vi "DMA-Ch.vi"(4 "DMATtoHOST":refnum<k21>="DMATtoHOST0", 6 "ProcessingFIFO":refnum<k21>="Processing0", 7 "IntermediateFIFO":refnum<k21>="FIFO0", 8 "Processing":bool, 10 "Source Name":refnum<k21>="100 MHz Clock", 11 "DMA number":i16) -> ()   [LabVIEW 2013]
uses:
  ctl.ctl
  StateControl.ctl
  <vilib>/Platform/TimedLoop/XDataNode/timing_clust.ctl
  <vilib>/Platform/TimedLoop/XDataNode/nitl_modes.ctl
  <vilib>/Platform/TimedLoop/XDataNode/wakeup.ctl
  N Channels.ctl
  <vilib>/rvi/Emulation/niFpgaSctlEmulationGetInTimedLoop.vi
  <vilib>/rvi/Emulation/niFpgaEmulationReportErrorSimple.vi
  <vilib>/rvi/Emulation/niFpgaGetClockAttributes.vi
  <vilib>/rvi/Emulation/niFpgaCriticalErrorInLSC.vi
  <vilib>/rvi/DataTransferAndStorage/Container/Common/niFpgaContainerExecOnDevCompGetState.vi
  <vilib>/rvi/FIFO/Fifo_Resource/nirvififoEmulationGetNumberOfElementsToReadFpgaImpl.vi
  <vilib>/rvi/DataTransferAndStorage/Container/Common/niFpgaContainerGetUniqueNameForEmu.vi
  <vilib>/rvi/interface/RandomDataEmulation/nirviRandomDataFPGAFIFO.vi
  <vilib>/rvi/interface/RandomDataEmulation/niFpgaRandomDataHandleErrors.vi
  <vilib>/rvi/eio/common/nirviEmuReportErrorAndStop.vi
  <vilib>/rvi/FIFO/Fifo_Resource/nirvififoEmulationReadFpgaImpl.vi
  <vilib>/rvi/FIFO/Fifo_Resource/nirvififoEmulationWriteFpgaImpl.vi
  <vilib>/rvi/Emulation/niFpgaProcessEmulError.vi
  GlobalReg.vi
  <vilib>/Platform/TimedLoop/XDataNode/XDataNode.xnode
  <vilib>/rvi/DataTransferAndStorage/Container/XNode/niFpgaContainer.xnode
  <vilib>/rvi/FIFO/Fifo_Resource/niFpgaFifoEmulationRefIn.vi
  <vilib>/rvi/interface/RandomDataEmulation/nirviRandomDataFpgaReadWriteTemplate.vi
  <vilib>/Platform/TimedLoop/XDataNode/XDNodeRunTimeDep.lvlib
panel:
  in  "Cluster in":T1
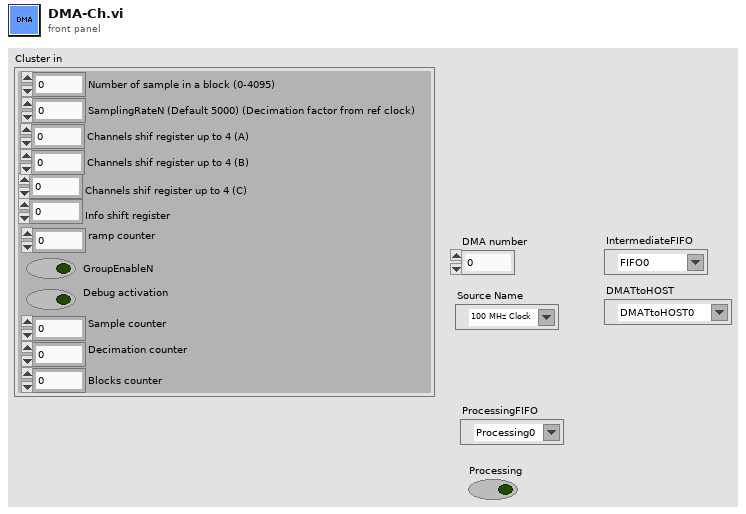
[diagram p1: front panel]
types:
  T1 = typedef "ctl.ctl" = cluster{"Number of sample in a block (0-4095)":u16, "SamplingRateN (Default 5000) (Decimation factor from ref clock)":u16, "Channels shif register up to 4 (A) ":u64, "Channels shif register up to 4 (B) ":u64, "Channels shif register up to 4 (C) ":u64, "Info shift register":u64, "ramp counter":i16, "GroupEnableN":bool, "Debug activation":bool, "Sample counter ":u64, "Decimation counter":u16, "Blocks counter":u16}
  T2 = typedef "StateControl.ctl" = enum16{"Idle", "Acq"}
  T3 = typedef "XDNodeRunTimeDep.lvlib/timing_clust.ctl" = cluster{"Expected End [f-1]":u64, "Actual End [f-1]":u64, "Finished Late? [f-1]":bool, "Expected End [i-1]":u64, "Actual End [i-1]":u64, "Finished Late? [i-1]":bool, "Expected Start [i]":u64, "Actual Start [i]":u64, "Expected Start [f]":u64, "Actual Start [f]":u64, "Source Name":string, "Structure Name":string, "Period":i64, "Deadline":i64, "Offset":i64, "Start":i64, "Priority":i32, "Timeout":i32, "Mode":T4, "Wakeup Reason":T5, "Error":errorcluster, "Source Type":string, "Secondary Source Type":string, "Global End Time":u64, "Global Start Time":u64, "Frame Duration":u64, "Iteration Duration":u64, "Assigned CPU":i32, "I/O Scan Engine Mode":u32}
  T4 = typedef "XDNodeRunTimeDep.lvlib/nitl_modes.ctl" = enum32{"No Change", "Process missed periods, maintain original phase", "Discard missed periods, maintain original phase", "Process missed periods, ignore original phase", "Discard missed periods, ignore original phase"}
  T5 = typedef "XDNodeRunTimeDep.lvlib/wakeup.ctl" = enum32{"Normal", "Aborted", "Asynchronous wakeup", "Timing source error", "Timed loop error", "Timeout"}
  T6 = typedef "N Channels.ctl" = enum16{"0 Channels", "1 Channels", "2 Channels", "3 Channels", "4 Channels", "5 Channels", "6 Channels", "7 Channels", "8 Channels", "9 Channels", "10 Channels", "11 Channels", "12 Channels"}
  T7 = cluster{u16, u16, u64, u64, u64, u64, i16, bool, bool, u64, u16, u16}
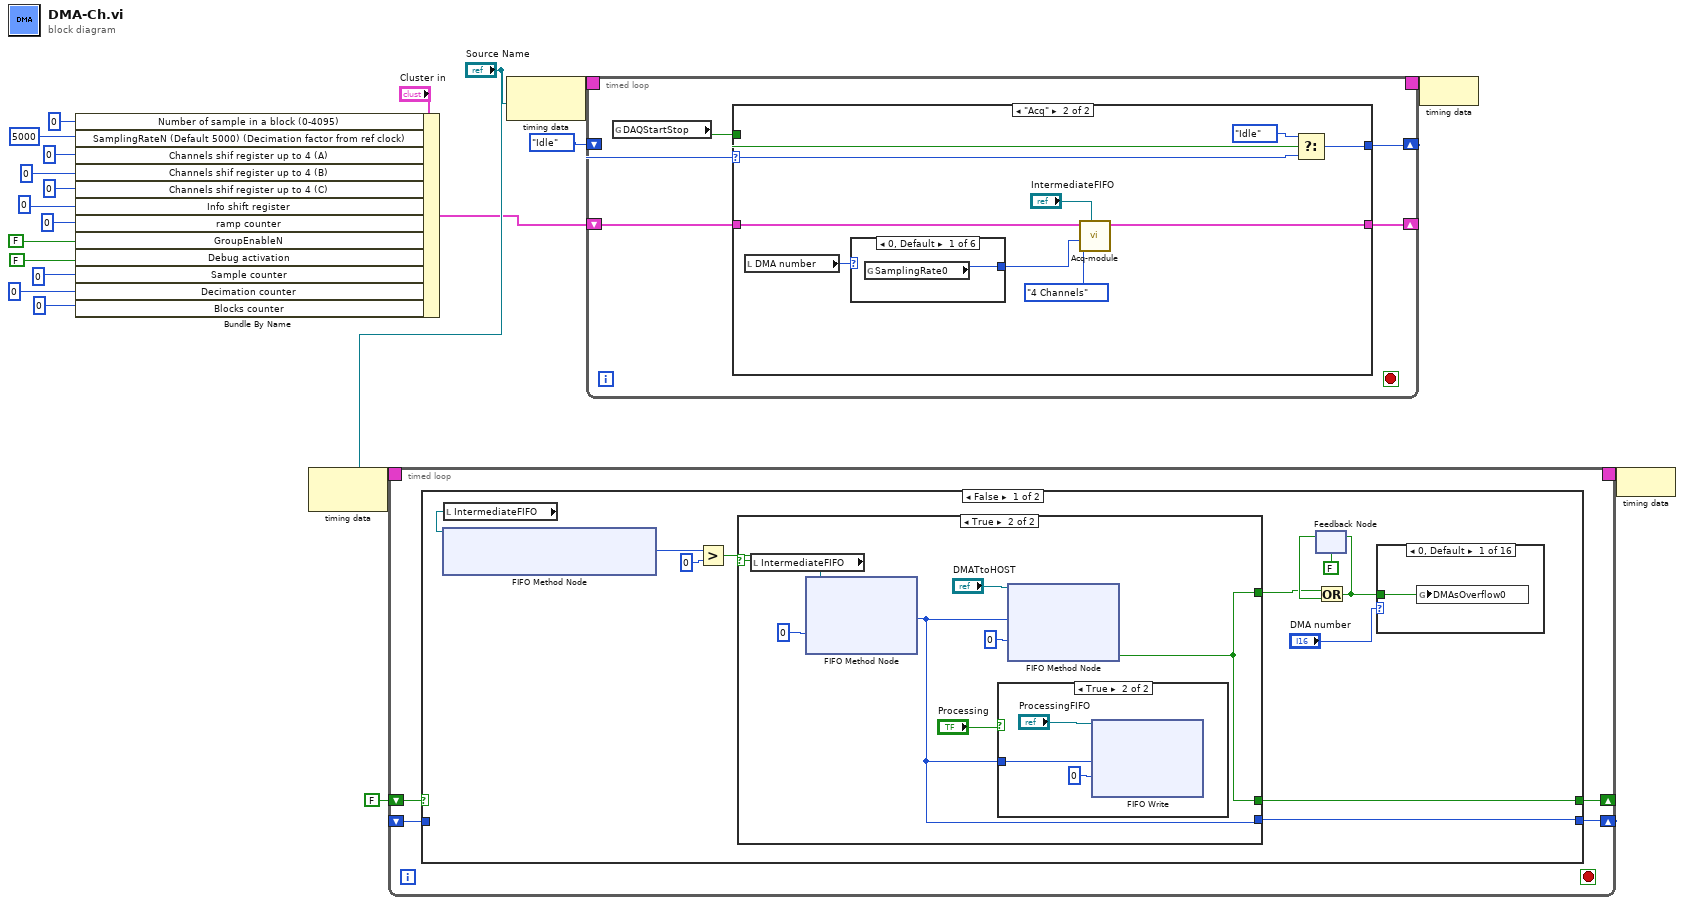
[diagram p0: block diagram]
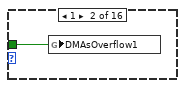
[diagram p2: hidden frame]
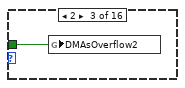
[diagram p3: hidden frame]
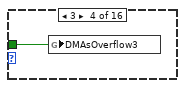
[diagram p4: hidden frame]
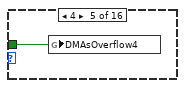
[diagram p5: hidden frame]
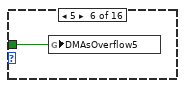
[diagram p6: hidden frame]
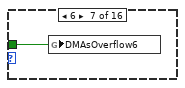
[diagram p7: hidden frame]
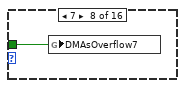
[diagram p8: hidden frame]
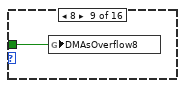
[diagram p9: hidden frame]
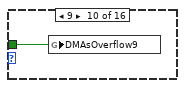
[diagram p10: hidden frame]
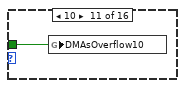
[diagram p11: hidden frame]
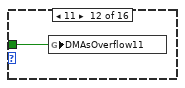
[diagram p12: hidden frame]
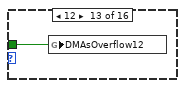
[diagram p13: hidden frame]
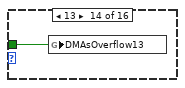
[diagram p14: hidden frame]
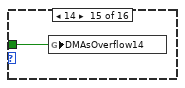
[diagram p15: hidden frame]
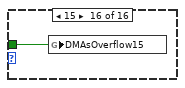
[diagram p16: hidden frame]
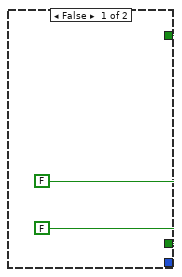
[diagram p17: hidden frame]
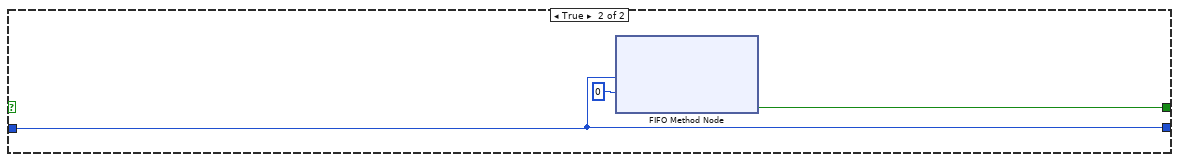
[diagram p19: hidden frame]
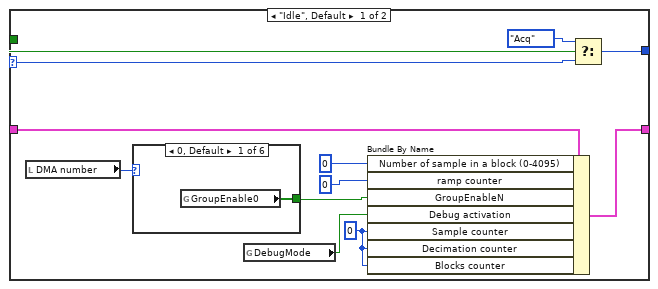
[diagram p20: hidden frame]
diagram:
  n1 = Bundle By Name(cluster="Cluster in", "Number of sample in a block (0-4095)"=u16 0 ("sample of block out"), "SamplingRateN (Default 5000) (Decimation factor from ref clock)"=u16 5000 ("FS1"), "Channels shif register up to 4 (A)"=u64 0, "Channels shif register up to 4 (B)"=u64 0, "Channels shif register up to 4 (C)"=u64 0, "Info shift register"=u64 0 ("Element"), "ramp counter"=i16 0, "GroupEnableN"=FALSE ("DMA1activation"), "Debug activation"=FALSE, "Sample counter"=u64 0 ("contador muestra"), "Decimation counter"=u16 0, "Blocks counter"=u16 0) -> (w1:T1)
  n2 = node-c288("Source Name") -> (w18:T3)
  n3 = timed-loop {
    timing: w18 -> [_]
    timing-out: [_] -> w17
    shift-right: [w25] -> _
    shift-left: FALSE ("Timed Out?") -> [w24]
    shift-right: [w23] -> _
    shift-left: _ -> [w22]
    stop <- _ stop-if-true
    n4 = case shown="False" w24 {
      tunnel: [w30 w66] -> w25
      tunnel: [w29 w65] -> w23
      tunnel: w22 -> [_ w65]
      frame False {
        n5 = local read "IntermediateFIFO"() -> (w26:refnum<k21>)
        n6 = xnode ("FIFO Method Node")("FIFO In"=w26) -> ("Number of Elements to Read"=w33:u32)  [unwired: 1 out]
        n7 = Greater?(x=w33, y=u32 0) -> (0:w31:bool)
        n8 = case shown="True" w31 {
          tunnel: [FALSE ("Timed Out?") w59] -> w34
          tunnel: [FALSE ("Timed Out?") w59] -> w30
          tunnel: [_ w57] -> w29
          frame False {
          }
          frame True {
            n9 = local read "IntermediateFIFO"() -> (w56:refnum<k21>)
            n10 = xnode ("FIFO Method Node")("Timeout"=0, "FIFO In"=w56) -> ("Element"=w57:u64)  [unwired: 2 out]
            n11 = case shown="True" "Processing" {
              tunnel: w57 -> [_ w63]
              frame False {
              }
              frame True {
                n12 = xnode ("FIFO Write")("Element"=w63, "Timeout"=0, "FIFO In"="ProcessingFIFO") -> ()  [unwired: 2 out]
              }
            }
            n13 = xnode ("FIFO Method Node")("Element"=w57, "Timeout"=0, "FIFO In"="DMATtoHOST") -> ("Timed Out?"=w59:bool)  [unwired: 1 out]
          }
        }
        n14 = feedback #1(FALSE) -> (w35:bool)
        n15 = Or(x=w34, y=w35) -> (x .or. y?=w27:bool)
        n16 = feedback-in #1(w27) -> ()
        n17 = case shown="0, Default" "DMA number" {
          tunnel: w27 -> [w37 w38 w39 w40 w41 w42 w43 w44 w45 w46 w47 w48 w49 w50 w51 w52]
          frame 0, Default {
            n18 = global write "GlobalReg.vi" "DMAsOverflow0"(w37) -> ()
          }
          frame 1 {
            n19 = global write "GlobalReg.vi" "DMAsOverflow1"(w38) -> ()
          }
          frame 2 {
            n20 = global write "GlobalReg.vi" "DMAsOverflow2"(w39) -> ()
          }
          frame 3 {
            n21 = global write "GlobalReg.vi" "DMAsOverflow3"(w40) -> ()
          }
          frame 4 {
            n22 = global write "GlobalReg.vi" "DMAsOverflow4"(w41) -> ()
          }
          frame 5 {
            n23 = global write "GlobalReg.vi" "DMAsOverflow5"(w42) -> ()
          }
          frame 6 {
            n24 = global write "GlobalReg.vi" "DMAsOverflow6"(w43) -> ()
          }
          frame 7 {
            n25 = global write "GlobalReg.vi" "DMAsOverflow7"(w44) -> ()
          }
          frame 8 {
            n26 = global write "GlobalReg.vi" "DMAsOverflow8"(w45) -> ()
          }
          frame 9 {
            n27 = global write "GlobalReg.vi" "DMAsOverflow9"(w46) -> ()
          }
          frame 10 {
            n28 = global write "GlobalReg.vi" "DMAsOverflow10"(w47) -> ()
          }
          frame 11 {
            n29 = global write "GlobalReg.vi" "DMAsOverflow11"(w48) -> ()
          }
          frame 12 {
            n30 = global write "GlobalReg.vi" "DMAsOverflow12"(w49) -> ()
          }
          frame 13 {
            n31 = global write "GlobalReg.vi" "DMAsOverflow13"(w50) -> ()
          }
          frame 14 {
            n32 = global write "GlobalReg.vi" "DMAsOverflow14"(w51) -> ()
          }
          frame 15 {
            n33 = global write "GlobalReg.vi" "DMAsOverflow15"(w52) -> ()
          }
        }
      }
      frame True {
        n34 = xnode ("FIFO Method Node")("Element"=w65, "Timeout"=0) -> ("Timed Out?"=w66:bool)  [unwired: 1 in, 1 out]
      }
    }
  }
  n35 = node-c288("Source Name") -> (w21:T3)
  n36 = timed-loop {
    timing: w21 -> [_]
    timing-out: [_] -> w20
    shift-right: [w73] -> _
    shift-left: StateControl."Idle" ("Enum") -> [w74]
    shift-right: [w70] -> _
    shift-left: w1 -> [w71]
    stop <- _ stop-if-true
    n37 = global read "GlobalReg.vi" "DAQStartStop"() -> (w72:bool)
    n38 = case shown="\"Acq\"" w74 {
      selector: w74 -> [w84 w101]
      tunnel: w72 -> [w86 w94]
      tunnel: [w83 w100] -> w73
      tunnel: w71 -> [w81 w96]
      tunnel: [w76 w95] -> w70
      frame "Idle", Default {
        w75 = i16 0
        n39 = local read "DMA number"() -> (w82:i16)
        n40 = case shown="0, Default" w82 {
          tunnel: [w87 w88 w89 w90 w91 w92] -> w77
          frame 0, Default {
            n41 = global read "GlobalReg.vi" "GroupEnable0"() -> (w87:bool)
          }
          frame 1 {
            n42 = global read "GlobalReg.vi" "GroupEnable1"() -> (w88:bool)
          }
          frame 2 {
            n43 = global read "GlobalReg.vi" "GroupEnable2"() -> (w89:bool)
          }
          frame 3 {
            n44 = global read "GlobalReg.vi" "GroupEnable3"() -> (w90:bool)
          }
          frame 4 {
            n45 = global read "GlobalReg.vi" "GroupEnable4"() -> (w91:bool)
          }
          frame 5 {
            n46 = global read "GlobalReg.vi" "GroupEnable5"() -> (w92:bool)
          }
        }
        n47 = global read "GlobalReg.vi" "DebugMode"() -> (w78:bool)
        n48 = Bundle By Name(cluster=w81, "Number of sample in a block (0-4095)"=u16 0, "ramp counter"=u64 0, "GroupEnableN"=w77, "Debug activation"=w78, "Sample counter"=w75, "Decimation counter"=w75, "Blocks counter"=w75) -> (w76:T1)
        n49 = Select(t=StateControl."Acq" ("Enum"), s=w86, f=w84) -> (s? t:f=w83:T2)
      }
      frame "Acq" {
        n50 = local read "DMA number"() -> (w99:i16)
        n51 = case shown="0, Default" w99 {
          tunnel: [w103 w104 w105 w106 w107 w108] -> w98
          frame 0, Default {
            n52 = global read "GlobalReg.vi" "SamplingRate0"() -> (w103:u16)
          }
          frame 1 {
            n53 = global read "GlobalReg.vi" "SamplingRate1"() -> (w104:u16)
          }
          frame 2 {
            n54 = global read "GlobalReg.vi" "SamplingRate2"() -> (w105:u16)
          }
          frame 3 {
            n55 = global read "GlobalReg.vi" "SamplingRate3"() -> (w106:u16)
          }
          frame 4 {
            n56 = global read "GlobalReg.vi" "SamplingRate4"() -> (w107:u16)
          }
          frame 5 {
            n57 = global read "GlobalReg.vi" "SamplingRate5"() -> (w108:u16)
          }
        }
        n58 = call "Acq-module.vi"("IntermediateFIFO"="IntermediateFIFO", "NumChannels"=N_Channels."4 Channels", "SamplingRate0"=w98, "Cluster in"=w96) -> ("cluster out"=w95:T7)  [unwired: 7 in]
        n59 = Select(t=StateControl."Idle" ("Enum"), s=w94, f=w101) -> (s? t:f=w100:T2)
      }
    }
  }
  n60 = node-c288(w20) -> ()
  n61 = node-c288(w17) -> ()
